vi "CSTK_Icon_Creator_Save.vi"(6 "image data":T1 caption="图像数据", 7 "路径字符":string, 8 "错误输入（无错误）":errorcluster, 10 "序号":i32, 11 "标题字符":string) -> (0 "错误输出":errorcluster)   [LabVIEW 2015, in "CSTK_Icon Creator.lvlib"]
uses:
  CSTK_Icon Creator.lvlib
  <vilib>/picture/picture.llb/imagedata.ctl
  <vilib>/Utility/sysdir.llb/System Directory Type.ctl
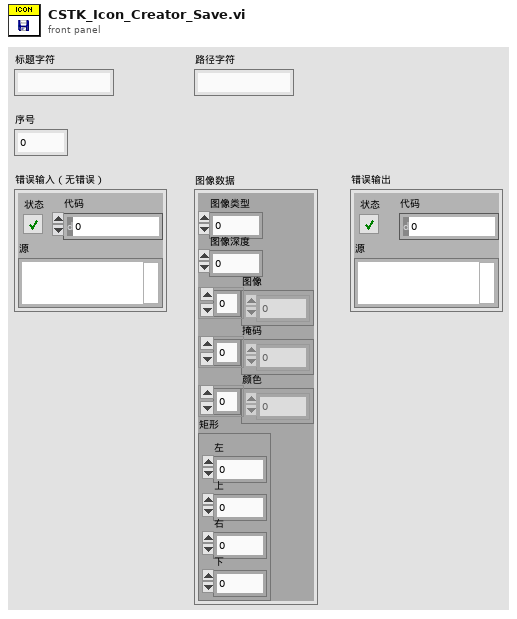
[diagram p1: front panel]
types:
  T1 = typedef "imagedata.ctl" = cluster{"image type":i32, "image depth":i32, "image":u8[], "mask":u8[], "colors":u32[], "Rectangle":cluster{"left":i16, "top":i16, "right":i16, "bottom":i16}}
  T2 = typedef "System Directory Type.ctl" = i32
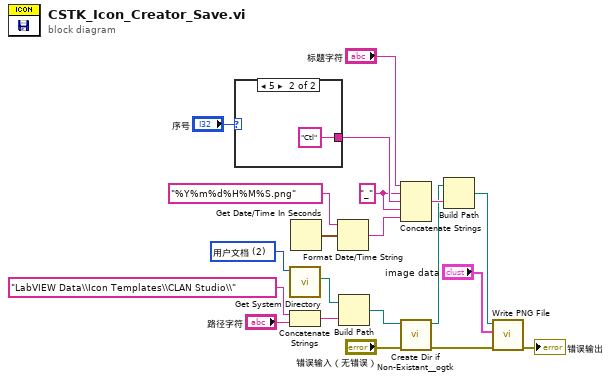
[diagram p0: block diagram]
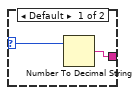
[diagram p2: hidden frame]
diagram:
  w5 = "_" ("字符串")
  w6 = T2 2 items=["用户目录"=0, "用户桌面"=1, "用户文档"=2, "用户应用程序数据"=3, "用户设置"=4, "用户临时目录"=5, "公共文档"=6, "公共应用程序数据"=7, "公共设置"=8, "公共缓存"=13, "系统核心库"=9, "系统安装库"=10, "应用程序文件"=11, "启动盘根目录"=12] ("system directory type")
  n1 = case shown="5" "序号" {
    selector: "序号" -> [w21 _]
    tunnel: [w22 "Ctl"] -> w15
    frame Default {
      n2 = Number To Decimal String(number=w21) -> (decimal integer string=w22:string)  [unwired: 1 in]
    }
    frame 5 {
    }
  }
  n3 = call <vilib>:"Get System Directory.vi"("system directory type"=w6) -> ("system directory"=w7:path)  [unwired: 10 in]
  n4 = Concatenate Strings("LabVIEW Data\\Icon Templates\\CLAN Studio\\" ("名称或相对路径"), "路径字符") -> (w10:string)
  n5 = Get Date/Time In Seconds() -> (seconds since 1Jan1904=w4:timestamp)
  n6 = Format Date/Time String(time format string (%c)="%Y%m%d%H%M%S.png" ("时间格式字符串(%c)"), seconds (now)=w4) -> (date/time string=w2:string)  [unwired: 1 in]
  n7 = Build Path(base path=w7, name or relative path=w10) -> (appended path=w9:path)
  n8 = Concatenate Strings("标题字符", w5, w15, w5, w2) -> (w16:string)
  n9 = call <userlib>:"Create Dir if Non-Existant__ogtk.vi"("error in (no error)"="错误输入（无错误）", "Directory Path"=w9) -> ("error out"=w19:errorcluster, "dup Directory Path"=w12:path)  [unwired: 7 in, 1 out]
  n10 = Build Path(base path=w12, name or relative path=w16) -> (appended path=w17:path)
  n11 = call <vilib>:"Write PNG File.vi"("error in (no error)"=w19, "image data"="image data", "path to PNG file"=w17) -> ("error out"=→"错误输出":errorcluster)  [unwired: 7 in, 1 out]
